vi "Allsel.vi"(7 "error in":errorcluster) -> (27 "error out":errorcluster)   [LabVIEW 2017]
uses:
  <vilib>/vision/NI_Vision_Development_Module.lvlib
panel:
  out "Shape Report (calibrated) 4":T1(array[cluster]) {"Score" format="%.2f"; "Centroid"."y" format="%.2f"; "Centroid"."x" format="%.2f"}
  out "Number of Matches 4":i32
  out "Shape Report (calibrated) 3":T1(array[cluster]) {"Score" format="%.2f"; "Centroid"."y" format="%.2f"; "Centroid"."x" format="%.2f"}
  out "Number of Matches 3":i32
  out "Shape Report (calibrated) 2":T1(array[cluster]) {"Score" format="%.2f"; "Centroid"."y" format="%.2f"; "Centroid"."x" format="%.2f"}
  out "Number of Matches 2":i32
  out "Shape Report (calibrated)":T1(array[cluster]) {"Score" format="%.2f"; "Centroid"."y" format="%.2f"; "Centroid"."x" format="%.2f"}
  out "Number of Matches":i32
  out "Image Out":T2(plugin-control)
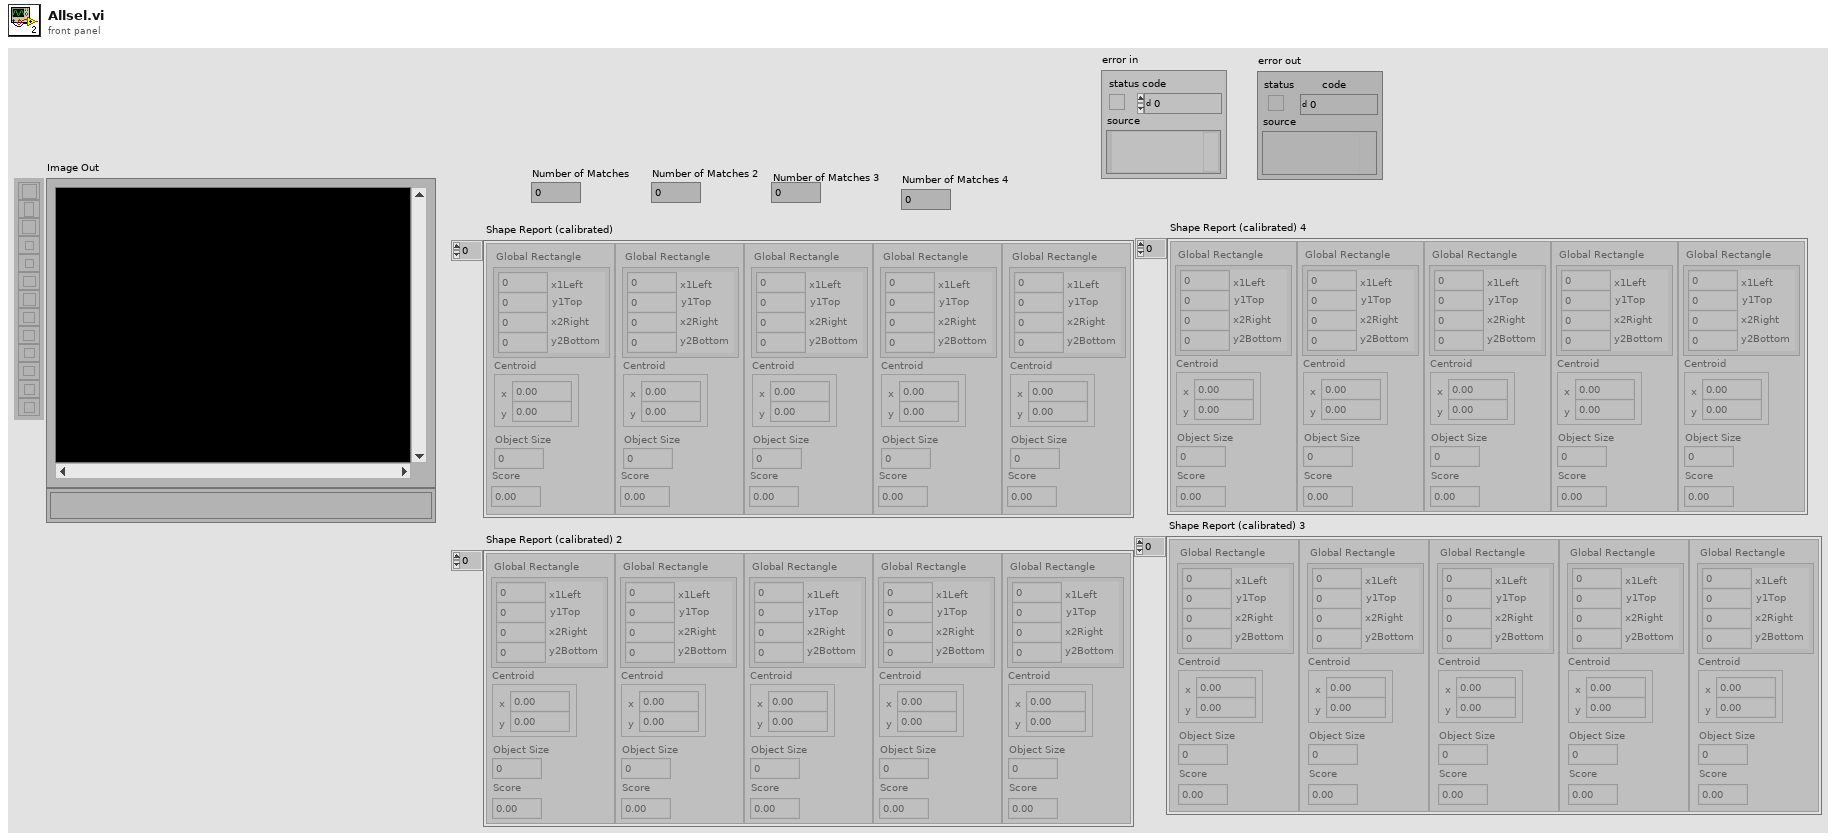
[diagram p1: front panel]
types:
  T1 = cluster{"Global Rectangle":cluster{"x1Left":i32, "y1Top":i32, "x2Right":i32, "y2Bottom":i32}, "Centroid":cluster{"x":sgl, "y":sgl}, "Object Size":u32, "Score":dbl}[]
  T2 = typedef "IMAQ Image.ctl" = refnum<image>
  T3 = typedef "Image Type" = u32
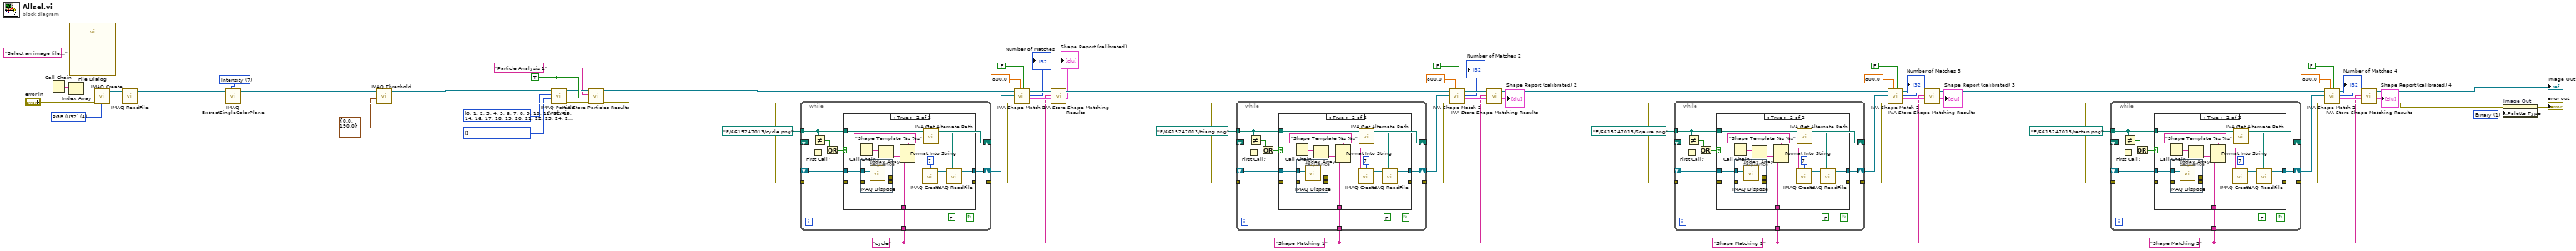
[diagram p0: block diagram]
diagram:
  w9 = u32 1 items=["Grayscale", "Binary", "Gradient", "Rainbow", "Temperature", "User Defined", "Binary 16 Bit", "Gradient 16 Bit", "Rainbow 16 Bit", "Temperature 16 Bit", "User Defined 16 Bit"] ("Palette Type")
  w12 = "Shape Matching 3" ("Step Name")
  w23 = "Shape Matching 2" ("Step Name")
  w34 = "Shape Matching 1" ("Step Name")
  w45 = "cycle" ("Step Name")
  w62 = i32[] [] items=["Center of Mass X", "Center of Mass Y", "First Pixel X", "First Pixel Y", "Bounding Rect Left", "Bounding Rect Top", "Bounding Rect Right", "Bounding Rect Bottom", "Max Feret Diameter Start X", "Max Feret Diameter Start Y", "Max Feret Diameter End X", "Max Feret Diameter End Y", "Max Horiz. Segment Length Left", "Max Horiz. Segment Length Right", "Max Horiz. Segment Length Row", "-", "Bounding Rect Width", "Bounding Rect Height", "Bounding Rect Diagonal", "Perimeter", "Convex Hull Perimeter", "Holes' Perimeter", "Max Feret Diameter", "Equivalent Ellipse Major Axis", "Equivalent Ellipse Minor Axis", "Equivalent Ellipse Minor Axis (Feret)", "Equivalent Rect Long Side", "Equivalent Rect Short Side", "Equivalent Rect Diagonal", "Equivalent Rect Short Side (Feret)", "Average Horiz. Segment Length", "Average Vert. Segment Length", "Hydraulic Radius", "Waddel Disk Diameter", "-", "Area", "Holes' Area", "Particle & Holes' Area", "Convex Hull Area", "Image Area", "-", "Number of Holes", "Number of Horiz. Segments", "Number of Vert. Segments", "-", "Orientation", "Max Feret Diameter Orientation", "-", "% Area/Image Area", "% Area/(Particle & Holes' Area)", "Ratio of Equivalent Ellipse Axes", "Ratio of Equivalent Rect Sides", "-", "Elongation Factor", "Compactness Factor", "Heywood Circularity Factor", "Type Factor", "-", "Sum X", "Sum Y", "Sum XX", "Sum XY", "Sum YY", "Sum XXX", "Sum XXY", "Sum XYY", "Sum YYY", "-", "Moment of Inertia XX", "Moment of Inertia XY", "Moment of Inertia YY", "Moment of Inertia XXX", "Moment of Inertia XXY", "Moment of Inertia XYY", "Moment of Inertia YYY", "Norm. Moment of Inertia XX", "Norm. Moment of Inertia XY", "Norm. Moment of Inertia YY", "Norm. Moment of Inertia XXX", "Norm. Moment of Inertia XXY", "Norm. Moment of Inertia XYY", "Norm. Moment of Inertia YYY", "Hu Moment 1", "Hu Moment 2", "Hu Moment 3", "Hu Moment 4", "Hu Moment 5", "Hu Moment 6", "Hu Moment 7"] ("Real-World Measurements")
  w63 = i32[] [0, 1, 2, 3, 4, 5, 6, 7, 8, 9, 10, 11, 12, 13, 14, 16, 17, 18, 19, 20, 21, 22, 23, 24, 25, 26, 27, 28, 29, 30, 31, 32, 33, 35, 36, 37, 38, 39, 41, 42, 43, 45, 46, 48, 49, 50, 51, 53, 54, 55, 56, 58, 59, 60, 61, 62, 63, 64, 65, 66, 68, 69, 70, 71, 72, 73, 74, 75, 76, 77, 78, 79, 80, 81, 82, 83, 84, 85, 86, 87, 88] items=["Center of Mass X", "Center of Mass Y", "First Pixel X", "First Pixel Y", "Bounding Rect Left", "Bounding Rect Top", "Bounding Rect Right", "Bounding Rect Bottom", "Max Feret Diameter Start X", "Max Feret Diameter Start Y", "Max Feret Diameter End X", "Max Feret Diameter End Y", "Max Horiz. Segment Length Left", "Max Horiz. Segment Length Right", "Max Horiz. Segment Length Row", "-", "Bounding Rect Width", "Bounding Rect Height", "Bounding Rect Diagonal", "Perimeter", "Convex Hull Perimeter", "Holes' Perimeter", "Max Feret Diameter", "Equivalent Ellipse Major Axis", "Equivalent Ellipse Minor Axis", "Equivalent Ellipse Minor Axis (Feret)", "Equivalent Rect Long Side", "Equivalent Rect Short Side", "Equivalent Rect Diagonal", "Equivalent Rect Short Side (Feret)", "Average Horiz. Segment Length", "Average Vert. Segment Length", "Hydraulic Radius", "Waddel Disk Diameter", "-", "Area", "Holes' Area", "Particle & Holes' Area", "Convex Hull Area", "Image Area", "-", "Number of Holes", "Number of Horiz. Segments", "Number of Vert. Segments", "-", "Orientation", "Max Feret Diameter Orientation", "-", "% Area/Image Area", "% Area/(Particle & Holes' Area)", "Ratio of Equivalent Ellipse Axes", "Ratio of Equivalent Rect Sides", "-", "Elongation Factor", "Compactness Factor", "Heywood Circularity Factor", "Type Factor", "-", "Sum X", "Sum Y", "Sum XX", "Sum XY", "Sum YY", "Sum XXX", "Sum XXY", "Sum XYY", "Sum YYY", "-", "Moment of Inertia XX", "Moment of Inertia XY", "Moment of Inertia YY", "Moment of Inertia XXX", "Moment of Inertia XXY", "Moment of Inertia XYY", "Moment of Inertia YYY", "Norm. Moment of Inertia XX", "Norm. Moment of Inertia XY", "Norm. Moment of Inertia YY", "Norm. Moment of Inertia XXX", "Norm. Moment of Inertia XXY", "Norm. Moment of Inertia XYY", "Norm. Moment of Inertia YYY", "Hu Moment 1", "Hu Moment 2", "Hu Moment 3", "Hu Moment 4", "Hu Moment 5", "Hu Moment 6", "Hu Moment 7"] ("Pixel Measurements")
  w60 = TRUE ("Connectivity 4/8 (8)")
  w69 = 7 items=["Red", "Green", "Blue", "Hue", "Saturation", "Luminance", "Value", "Intensity"] ("Color Plane")
  w70 = T3 4 items=["Grayscale (U8)", "Grayscale (I16)", "Grayscale (SGL)", "Complex (CSG)", "RGB (U32)", "HSL (U32)", "RGB (U64)", "Grayscale (U16)"] ("Image Type")
  n1 = Call Chain() -> (call chain=w74:string[])
  n2 = Index Array(array=w74) -> (element=w73:string)  [unwired: 1 in]
  n3 = call "File Dialog"("prompt"="Select an image file...") -> ("selected path"=w71:path)  [unwired: 6 in, 8 out]
  n4 = call "IMAQ Create"("Image Name"=w73, "Image Type"=w70, "error in (no error)"="error in") -> ("New Image"=w77:T2, "error out"=w76:errorcluster)  [unwired: 1 in, 1 out]
  n5 = call "IMAQ ReadFile"("File Path"=w71, "error in (no error)"=w76, "Image"=w77) -> ("error out"=w78:errorcluster, "Image Out"=w68:T2)  [unwired: 2 in, 5 out]
  n6 = call "IMAQ ExtractSingleColorPlane"("Color Plane"=w69, "error in (no error)"=w78, "Image Src"=w68) -> ("error out"=w67:errorcluster, "Image Dst Out"=w65:T2)  [unwired: 1 in, 6 out]
  n7 = call "IMAQ Threshold"("error in (no error)"=w67, "Range"=cluster{"Lower value":sgl, "Upper value":sgl} {"Lower value"=0.0, "Upper value"=190.0}, "Image Src"=w65) -> ("error out"=w64:errorcluster, "Image Dst Out"=w61:T2)  [unwired: 3 in, 4 out]
  n8 = call "IMAQ Particle Analysis"("Connectivity 4/8 (8)"=w60, "error in (no error)"=w64, "Real-World Measurements"=w62, "Pixel Measurements"=w63, "Image"=w61) -> ("error out"=w57:errorcluster, "Image Out (duplicate)"=w59:T2)  [unwired: 5 out]
  n9 = call <vilib>:"IVA Store Particles Results.vi"("error in (no error)"=w57, "Connectivity 4/8 (8)"=w60, "Step Name"="Particle Analysis 1", "Image in"=w59) -> ("error out"=w56:errorcluster, "Image dup"=w53:T2)  [unwired: 6 out]
  n10 = while {
    shift-right: [w89] -> w46
    shift-left: _ -> [w88]
    tunnel: [w86] -> w47
    tunnel: w56 -> [w85]
    tunnel: path "E:/6615247013/cycle.png" ("Template Path") -> [w83]
    tunnel: w45 -> [w84]
    shift-right: [w83] -> _
    shift-left: _ -> [w82]
    stop <- FALSE continue-if-true
    n11 = First Call?() -> (First Call?: T/F=w81:bool)
    n12 = Not Equal?(x=w83, y=w82) -> (x != y?=w80:bool)
    n13 = Or(x=w80, y=w81) -> (x .or. y?=w79:bool)
    n14 = case shown="True" w79 {
      tunnel: [w91 w103] -> w89
      tunnel: w88 -> [w91 w94]
      tunnel: [w90 w101] -> w86
      tunnel: w85 -> [w90 w93]
      tunnel: w83 -> [_ w96]
      tunnel: w84 -> [_ w97]
      frame False {
      }
      frame True {
        n15 = Call Chain() -> (call chain=w99:string[])
        n16 = stacked-sequence {
          tunnel: w94 -> [w109]
          tunnel: w93 -> [w108]
          tunnel: [w108] -> w92
          tunnel: [w107] -> _
          frame #0 {
            n17 = call "IMAQ Dispose"("Image"=w109) -> ("error out"=w107:errorcluster)  [unwired: 2 in, 3 out]
          }
        }
        n18 = Index Array(array=w99) -> (element=w98:string)  [unwired: 1 in]
        n19 = Format Into String(format string="Shape Template %s %s" ("Image Name"), w98, w97) -> (resulting string=w106:string)  [unwired: 2 in, 1 out]
        n20 = call "IMAQ Create"("Border Size"=7, "Image Name"=w106, "error in (no error)"=w92) -> ("New Image"=w104:T2, "error out"=w102:errorcluster)  [unwired: 1 in, 1 out]
        n21 = call <vilib>:"IVA Get Alternate Path.vi"("Path In"=w96) -> ("Path Out"=w95:path)  [unwired: 10 out]
        n22 = call "IMAQ ReadFile"("File Path"=w95, "error in (no error)"=w102, "Image"=w104) -> ("error out"=w101:errorcluster, "Image Out"=w103:T2)  [unwired: 2 in, 5 out]
      }
    }
  }
  n23 = call <vilib>:"IVA Shape Match 2.vi"("Scale Invariance"=FALSE, "Minimal Score"=800.0, "error in (no error)"=w47, "Template"=w46, "Image Src"=w53) -> ("error out"=w52:errorcluster, "Shape Report"=w50:T1, "Number of Matches"=→"Number of Matches":i32, "Image Out"=w49:T2)  [unwired: 3 out]
  n24 = call <vilib>:"IVA Store Shape Matching Results.vi"("error in (no error)"=w52, "Shape Report"=w50, "Step Name"=w45, "Image in"=w49) -> ("error out"=w51:errorcluster, "Shape Report (calibrated)"=→"Shape Report (calibrated)":T1, "Image dup"=w42:T2)  [unwired: 5 out]
  n25 = while {
    shift-right: [w120] -> w35
    shift-left: _ -> [w119]
    tunnel: [w117] -> w36
    tunnel: w51 -> [w116]
    tunnel: path "E:/6615247013/triang.png" ("Template Path") -> [w114]
    tunnel: w34 -> [w115]
    shift-right: [w114] -> _
    shift-left: _ -> [w113]
    stop <- FALSE continue-if-true
    n26 = First Call?() -> (First Call?: T/F=w112:bool)
    n27 = Not Equal?(x=w114, y=w113) -> (x != y?=w111:bool)
    n28 = Or(x=w111, y=w112) -> (x .or. y?=w110:bool)
    n29 = case shown="True" w110 {
      tunnel: [w122 w134] -> w120
      tunnel: w119 -> [w122 w125]
      tunnel: [w121 w132] -> w117
      tunnel: w116 -> [w121 w124]
      tunnel: w114 -> [_ w127]
      tunnel: w115 -> [_ w128]
      frame False {
      }
      frame True {
        n30 = Call Chain() -> (call chain=w130:string[])
        n31 = stacked-sequence {
          tunnel: w125 -> [w140]
          tunnel: w124 -> [w139]
          tunnel: [w139] -> w123
          tunnel: [w138] -> _
          frame #0 {
            n32 = call "IMAQ Dispose"("Image"=w140) -> ("error out"=w138:errorcluster)  [unwired: 2 in, 3 out]
          }
        }
        n33 = Index Array(array=w130) -> (element=w129:string)  [unwired: 1 in]
        n34 = Format Into String(format string="Shape Template %s %s" ("Image Name"), w129, w128) -> (resulting string=w137:string)  [unwired: 2 in, 1 out]
        n35 = call "IMAQ Create"("Border Size"=7, "Image Name"=w137, "error in (no error)"=w123) -> ("New Image"=w135:T2, "error out"=w133:errorcluster)  [unwired: 1 in, 1 out]
        n36 = call <vilib>:"IVA Get Alternate Path.vi"("Path In"=w127) -> ("Path Out"=w126:path)  [unwired: 10 out]
        n37 = call "IMAQ ReadFile"("File Path"=w126, "error in (no error)"=w133, "Image"=w135) -> ("error out"=w132:errorcluster, "Image Out"=w134:T2)  [unwired: 2 in, 5 out]
      }
    }
  }
  n38 = call <vilib>:"IVA Shape Match 2.vi"("Scale Invariance"=FALSE, "Minimal Score"=800.0, "error in (no error)"=w36, "Template"=w35, "Image Src"=w42) -> ("error out"=w41:errorcluster, "Shape Report"=w39:T1, "Number of Matches"=→"Number of Matches 2":i32, "Image Out"=w38:T2)  [unwired: 3 out]
  n39 = call <vilib>:"IVA Store Shape Matching Results.vi"("error in (no error)"=w41, "Shape Report"=w39, "Step Name"=w34, "Image in"=w38) -> ("error out"=w40:errorcluster, "Shape Report (calibrated)"=→"Shape Report (calibrated) 2":T1, "Image dup"=w31:T2)  [unwired: 5 out]
  n40 = while {
    shift-right: [w151] -> w24
    shift-left: _ -> [w150]
    tunnel: [w148] -> w25
    tunnel: w40 -> [w147]
    tunnel: path "E:/6615247013/Sqaure.png" ("Template Path") -> [w145]
    tunnel: w23 -> [w146]
    shift-right: [w145] -> _
    shift-left: _ -> [w144]
    stop <- FALSE continue-if-true
    n41 = First Call?() -> (First Call?: T/F=w143:bool)
    n42 = Not Equal?(x=w145, y=w144) -> (x != y?=w142:bool)
    n43 = Or(x=w142, y=w143) -> (x .or. y?=w141:bool)
    n44 = case shown="True" w141 {
      tunnel: [w153 w165] -> w151
      tunnel: w150 -> [w153 w156]
      tunnel: [w152 w163] -> w148
      tunnel: w147 -> [w152 w155]
      tunnel: w145 -> [_ w158]
      tunnel: w146 -> [_ w159]
      frame False {
      }
      frame True {
        n45 = Call Chain() -> (call chain=w161:string[])
        n46 = stacked-sequence {
          tunnel: w156 -> [w171]
          tunnel: w155 -> [w170]
          tunnel: [w170] -> w154
          tunnel: [w169] -> _
          frame #0 {
            n47 = call "IMAQ Dispose"("Image"=w171) -> ("error out"=w169:errorcluster)  [unwired: 2 in, 3 out]
          }
        }
        n48 = Index Array(array=w161) -> (element=w160:string)  [unwired: 1 in]
        n49 = Format Into String(format string="Shape Template %s %s" ("Image Name"), w160, w159) -> (resulting string=w168:string)  [unwired: 2 in, 1 out]
        n50 = call "IMAQ Create"("Border Size"=7, "Image Name"=w168, "error in (no error)"=w154) -> ("New Image"=w166:T2, "error out"=w164:errorcluster)  [unwired: 1 in, 1 out]
        n51 = call <vilib>:"IVA Get Alternate Path.vi"("Path In"=w158) -> ("Path Out"=w157:path)  [unwired: 10 out]
        n52 = call "IMAQ ReadFile"("File Path"=w157, "error in (no error)"=w164, "Image"=w166) -> ("error out"=w163:errorcluster, "Image Out"=w165:T2)  [unwired: 2 in, 5 out]
      }
    }
  }
  n53 = call <vilib>:"IVA Shape Match 2.vi"("Scale Invariance"=FALSE, "Minimal Score"=800.0, "error in (no error)"=w25, "Template"=w24, "Image Src"=w31) -> ("error out"=w30:errorcluster, "Shape Report"=w28:T1, "Number of Matches"=→"Number of Matches 3":i32, "Image Out"=w27:T2)  [unwired: 3 out]
  n54 = call <vilib>:"IVA Store Shape Matching Results.vi"("error in (no error)"=w30, "Shape Report"=w28, "Step Name"=w23, "Image in"=w27) -> ("error out"=w29:errorcluster, "Shape Report (calibrated)"=→"Shape Report (calibrated) 3":T1, "Image dup"=w20:T2)  [unwired: 5 out]
  n55 = while {
    shift-right: [w182] -> w13
    shift-left: _ -> [w181]
    tunnel: [w179] -> w14
    tunnel: w29 -> [w178]
    tunnel: path "E:/6615247013/rectan.png" ("Template Path") -> [w176]
    tunnel: w12 -> [w177]
    shift-right: [w176] -> _
    shift-left: _ -> [w175]
    stop <- FALSE continue-if-true
    n56 = First Call?() -> (First Call?: T/F=w174:bool)
    n57 = Not Equal?(x=w176, y=w175) -> (x != y?=w173:bool)
    n58 = Or(x=w173, y=w174) -> (x .or. y?=w172:bool)
    n59 = case shown="True" w172 {
      tunnel: [w184 w196] -> w182
      tunnel: w181 -> [w184 w187]
      tunnel: [w183 w194] -> w179
      tunnel: w178 -> [w183 w186]
      tunnel: w176 -> [_ w189]
      tunnel: w177 -> [_ w190]
      frame False {
      }
      frame True {
        n60 = Call Chain() -> (call chain=w192:string[])
        n61 = stacked-sequence {
          tunnel: w187 -> [w202]
          tunnel: w186 -> [w201]
          tunnel: [w201] -> w185
          tunnel: [w200] -> _
          frame #0 {
            n62 = call "IMAQ Dispose"("Image"=w202) -> ("error out"=w200:errorcluster)  [unwired: 2 in, 3 out]
          }
        }
        n63 = Index Array(array=w192) -> (element=w191:string)  [unwired: 1 in]
        n64 = Format Into String(format string="Shape Template %s %s" ("Image Name"), w191, w190) -> (resulting string=w199:string)  [unwired: 2 in, 1 out]
        n65 = call "IMAQ Create"("Border Size"=7, "Image Name"=w199, "error in (no error)"=w185) -> ("New Image"=w197:T2, "error out"=w195:errorcluster)  [unwired: 1 in, 1 out]
        n66 = call <vilib>:"IVA Get Alternate Path.vi"("Path In"=w189) -> ("Path Out"=w188:path)  [unwired: 10 out]
        n67 = call "IMAQ ReadFile"("File Path"=w188, "error in (no error)"=w195, "Image"=w197) -> ("error out"=w194:errorcluster, "Image Out"=w196:T2)  [unwired: 2 in, 5 out]
      }
    }
  }
  n68 = call <vilib>:"IVA Shape Match 2.vi"("Scale Invariance"=FALSE, "Minimal Score"=800.0, "error in (no error)"=w14, "Template"=w13, "Image Src"=w20) -> ("error out"=w19:errorcluster, "Shape Report"=w17:T1, "Number of Matches"=→"Number of Matches 4":i32, "Image Out"=w16:T2)  [unwired: 3 out]
  n69 = call <vilib>:"IVA Store Shape Matching Results.vi"("error in (no error)"=w19, "Shape Report"=w17, "Step Name"=w12, "Image in"=w16) -> ("error out"=w18:errorcluster, "Shape Report (calibrated)"=→"Shape Report (calibrated) 4":T1, "Image dup"=→"Image Out":T2)  [unwired: 5 out]
  n70 = property on="Image Out" class="ImageControl"(error in=w18, "Palette:Palette Type"=w9) -> (error out=→"error out":errorcluster)  [unwired: 1 in, 1 out]
